vi "Mass Compile.vi"(11 "WebView2 Updater in":refnum<class "WebView2 Updater.lvclass">) -> (0 "error out":errorcluster)   [LabVIEW 2020, in "WebView2 Updater.lvclass"]
uses:
  WebView2 Updater.lvclass
  WebView2 Updater.lvclass/WebView2 Updater.ctl
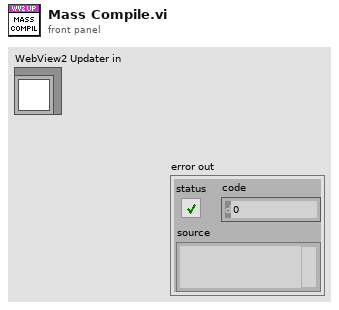
[diagram p1: front panel]
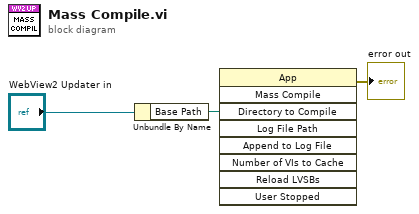
[diagram p0: block diagram]
diagram:
  n1 = Unbundle By Name("WebView2 Updater in") -> ("Base Path"=w3:path)
  n2 = invoke class="App" method="Mass Compile"("Directory to Compile"=w3) -> (error out=→"error out":errorcluster)  [unwired: 8 in, 8 out]
